vi "(SubVI) Calculate Xbd from QPD using 7th order PolyFit.vi"(4 "yr (V)":dbl, 5 "cr (um)":dbl, 7 "file path (dialog if empty)":path, 8 "Stage Position (um)":dbl[](array[numeric]), 9 "QPD Signal (V)":dbl[](array[numeric])) -> (2 "Xst (nm)":dbl[](array[numeric]), 3 "Xbead (nm)":dbl[](array[numeric]))   [LabVIEW 2014]
uses:
  <vilib>/Utility/file.llb/Read From Spreadsheet File (DBL).vi
  <vilib>/Analysis/polynomials.llb/Scalar Polynomial Evaluation (DBL).vi
  <vilib>/Analysis/NI_AALPro.lvlib
panel:
  out "XY Graph":cluster{dbl[], "Best Polynomial Fit":dbl[]}[](graph)
  out "stage center ,r=0":dbl
  out "Stage Max to min":dbl[](array[numeric])
  out "QPD Max to min":dbl[](array[numeric])
  out "Polynomial Coefficients":dbl[](array[numeric])
  out "Best Polynomial Fit":dbl[](array[numeric])
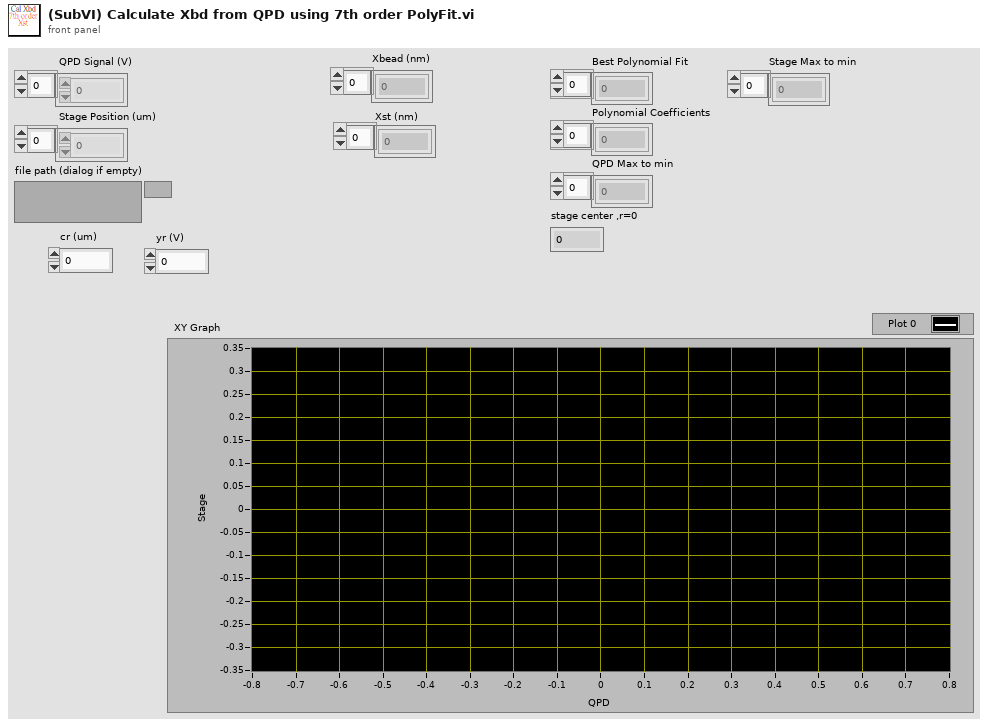
[diagram p1: front panel]
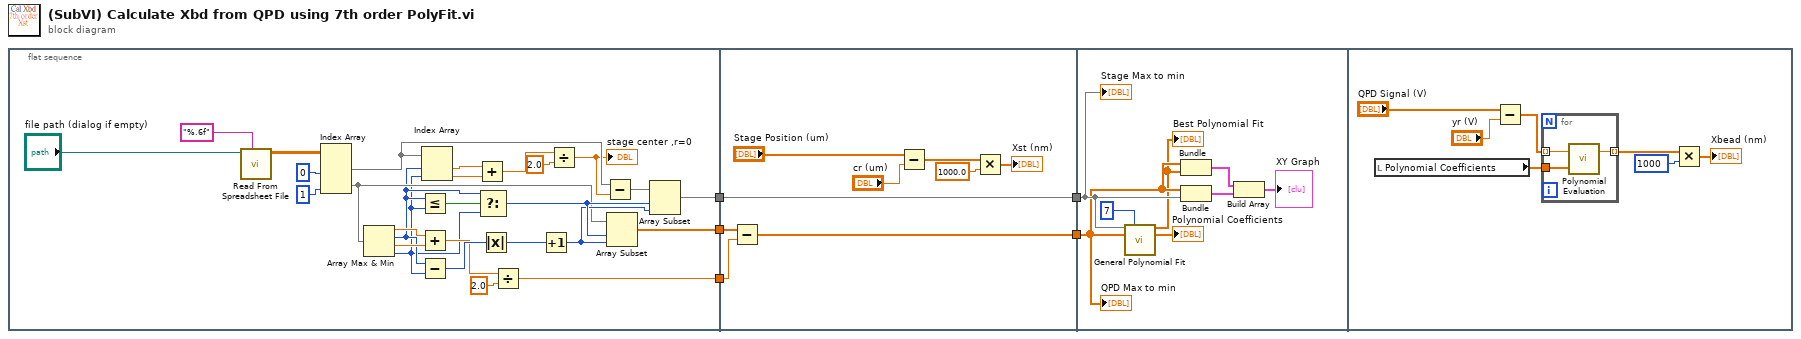
[diagram p0: block diagram]
diagram:
  n1 = flat-sequence {
    tunnel: [w29] -> w5
    tunnel: [w26] -> w3
    tunnel: [w21] -> w1
    tunnel: w5 -> [w41]
    tunnel: [w39] -> w4
    tunnel: w3 -> [w38]
    tunnel: [w38] -> w2
    tunnel: w1 -> [w40]
    tunnel: w4 -> [w46]
    tunnel: w2 -> [w47]
    frame #0 {
      n2 = call-poly <vilib>:"Read From Spreadsheet File.vi"("format (%.3f)"="%.6f", "file path (dialog if empty)"="file path (dialog if empty)") -> ("all rows"=w18:dbl[][])  [unwired: 5 in, 4 out]
      n3 = Index Array(array=w18, index (col) #1=0 ("disabled index (col)"), index (col) #2=1 ("disabled index (col)")) -> (element #1=w8:dbl[], element #2=w15:dbl[])  [unwired: 2 in]
      n4 = Array Max & Min(array=w15) -> (max value=w25:dbl, max index (indices)=w14:i32, min value=w24:dbl, min index (indices)=w13:i32)
      n5 = Less Or Equal?(x=w14, y=w13) -> (x <= y?=w32:bool)
      n6 = Add(x=w25, y=w24) -> (x+y=w23:dbl)
      n7 = Subtract(x=w14, y=w13) -> (x-y=w31:i32)
      n8 = Index Array(array=w8, index #1=w14, index #2=w13) -> (element #1=w12:dbl, element #2=w11:dbl)
      n9 = Add(x=w12, y=w11) -> (x+y=w9:dbl)
      n10 = Select(t=w14, s=w32, f=w13) -> (s? t:f=w28:i32)
      n11 = Absolute Value(x=w31) -> (abs(x)=w30:i32)
      n12 = Divide(x=w23, y=2.0) -> (x/y=w21:dbl)
      n13 = Increment(x=w30) -> (x+1=w27:i32)
      n14 = Divide(x=w9, y=2.0) -> (x/y=w7:dbl)
      "stage center ,r=0" <- w7
      n15 = Subtract(x=w8, y=w7) -> (x-y=w6:dbl[])
      n16 = Array Subset(array=w15, index=w28, length=w27) -> (w29:dbl[])
      n17 = Array Subset(array=w6, index=w28, length=w27) -> (w26:dbl[])
    }
    frame #1 {
      n18 = Subtract(x=w41, y=w40) -> (x-y=w39:dbl[])
      n19 = Subtract(x="Stage Position (um)", y="cr (um)") -> (x-y=w36:dbl[])
      n20 = Multiply(x=w36, y=1000.0) -> (x*y=→"Xst (nm)":dbl[])
    }
    frame #2 {
      n21 = call <vilib>:"General Polynomial Fit.vi"("Y"=w47, "polynomial order"=7, "X"=w46) -> ("Best Polynomial Fit"=w45:dbl[], "Polynomial Coefficients"=→"Polynomial Coefficients":dbl[])  [unwired: 9 in, 2 out]
      "Best Polynomial Fit" <- w45
      n22 = Bundle(w46, "Best Polynomial Fit"=w45) -> (w43:cluster{dbl[], "Best Polynomial Fit":dbl[]})  [unwired: 1 in]
      n23 = Bundle(w46, w47) -> (w44:cluster{dbl[], dbl[]})  [unwired: 1 in]
      n24 = Build Array(w43, w44) -> (→"XY Graph":cluster{dbl[], "Best Polynomial Fit":dbl[]}[])
      "QPD Max to min" <- w46
      "Stage Max to min" <- w47
    }
    frame #3 {
      n25 = local read "Polynomial Coefficients"() -> (w56:dbl[])
      n26 = Subtract(x="QPD Signal (V)", y="yr (V)") -> (x-y=w53:dbl[])
      n27 = for {
        tunnel: w53 -> [w59] mode=indexing
        tunnel: w56 -> [w58]
        tunnel: [w57] -> w52 mode=indexing
        n28 = call-poly <vilib>:"Polynomial Evaluation.vi"("P(x)"=w58, "a"=w59) -> ("P(a)"=w57:dbl)  [unwired: 1 out]
      }
      n29 = Multiply(x=w52, y=1000 ("P(a)")) -> (x*y=→"Xbead (nm)":dbl[])
    }
  }
